vi "GetQualifiedName.vi"(8 "error in (no error)":errorcluster, 10 "separator (dot)":string caption="separator", 11 "SMO":refnum<class "SMO.lvclass">) -> (0 "error out":errorcluster, 2 "Qualified Name":string, 3 "SMO out":refnum<class "SMO.lvclass">)   [LabVIEW 2021, in "smo.lvlib" / "SMO.lvclass"]
uses:
  SMO.lvclass
  SMO.lvclass/SMO.ctl
panel:
  # "For instructions on how to use the JKI State Machine Objects, examples and video tutorials, visit:\nhttp://jki.net/state-machine-objects/\n\nJKI State Machine Objects™\nhttp://jki.net/state-machine-objects/\nCopyright (C) 2005-2015, JKI <info@jki.net>\nALL RIGHTS RESERVED"
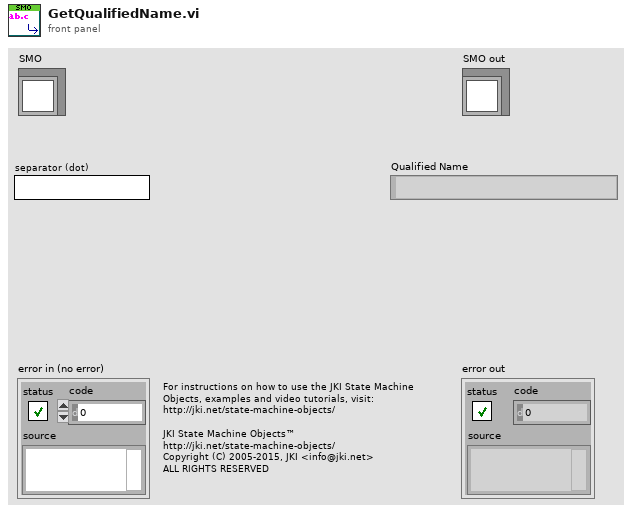
[diagram p1: front panel]
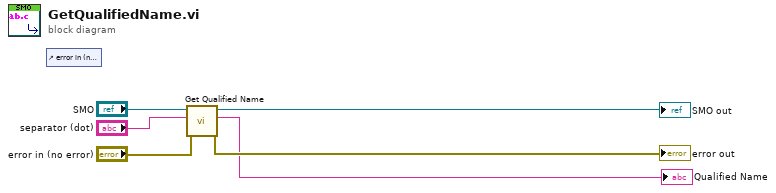
[diagram p0: block diagram]
diagram:
  n1 = control-ref of="error in (no error)"() -> ()  [unwired: 1 out]
  n2 = call "Get Qualified Name.vi"("error in (no error)"="error in (no error)", "separator (dot)"="separator (dot)", "SMO"="SMO") -> ("error out"=→"error out":errorcluster, "Qualified Name"=→"Qualified Name":string, "SMO out"=→"SMO out":refnum<class "SMO.lvclass">)  [unwired: 5 in, 1 out]
